vi "User mangement.vi"() -> ()   [LabVIEW 2017]
uses:
  <vilib>/Utility/error.llb/DialogType.ctl
  <vilib>/addons/database/Connection.llb/DB Tools Open Connec (Path).vi
  <vilib>/addons/database/NI_Database_API.lvlib
panel:
  in  "NEW":bool
  in  "DELETE":bool
  out "error out":errorcluster
  in  "error in (no error)":errorcluster
  in  "EXIT":bool
  in  "SAVE":bool
  in  "Authority":string(combo)
  in  "re_enter password":string
  in  "Password":string
  in  "NAME":string(combo)
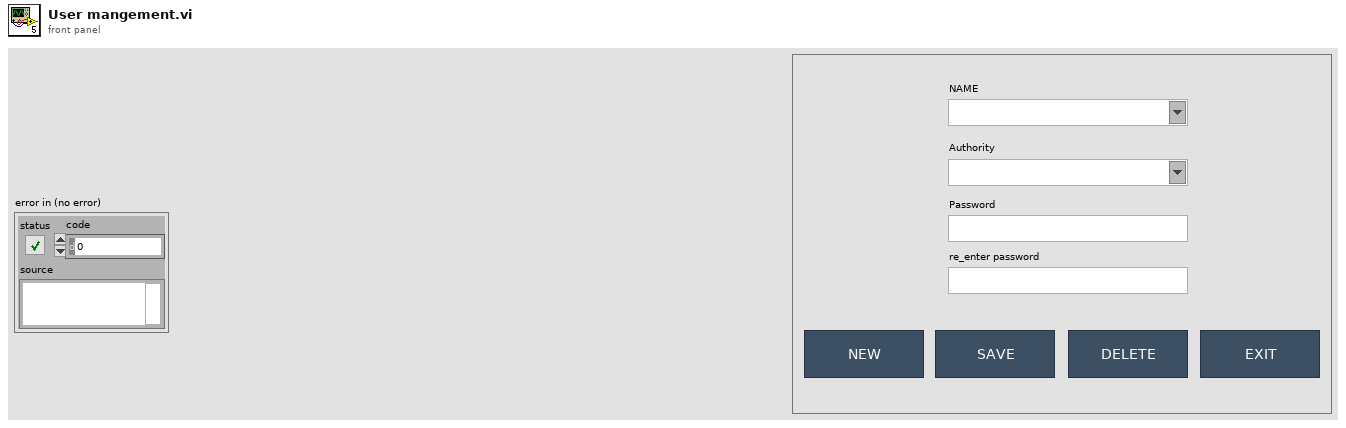
[diagram p1: front panel]
types:
  T1 = typedef "DialogType.ctl" = u16
  T2 = typedef "NI_Database_API.lvlib/Conn ObjectReference.ctl" = refnum<k1>
  T3 = cluster{"NAME":string, "Authority":string, "Password":string, "re_enter password":string}
  T4 = enum32{"invalid app kind", "Development System", "Run Time System", "Student Edition", "Embedded LabVIEW", "Evaluation", "Custom"}
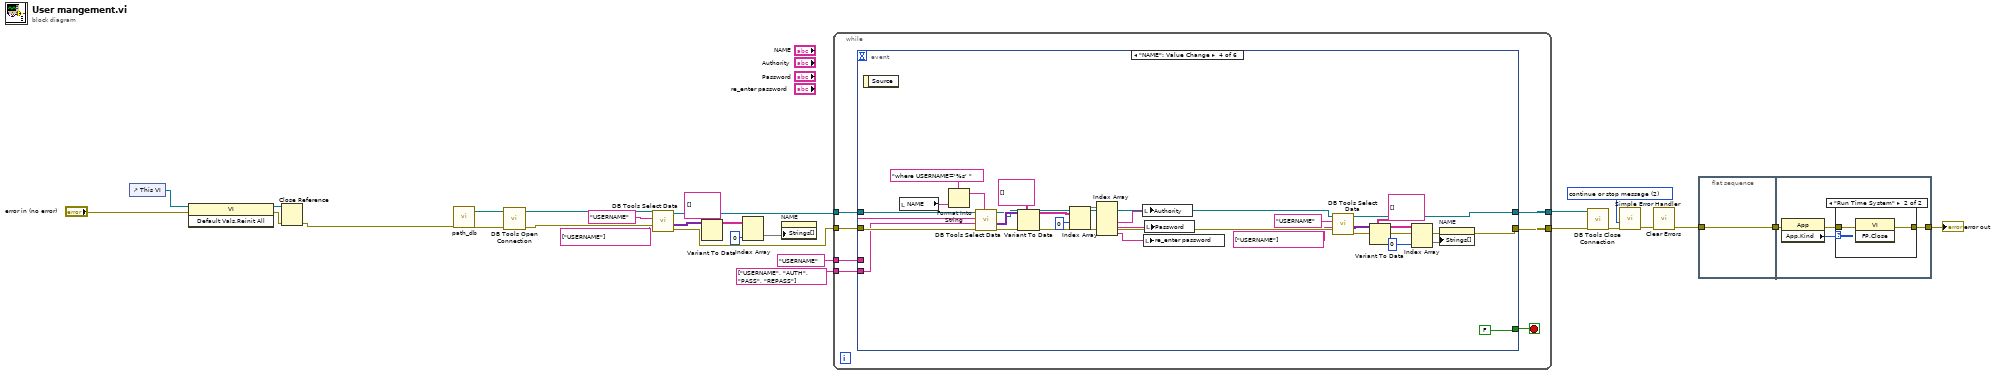
[diagram p0: block diagram]
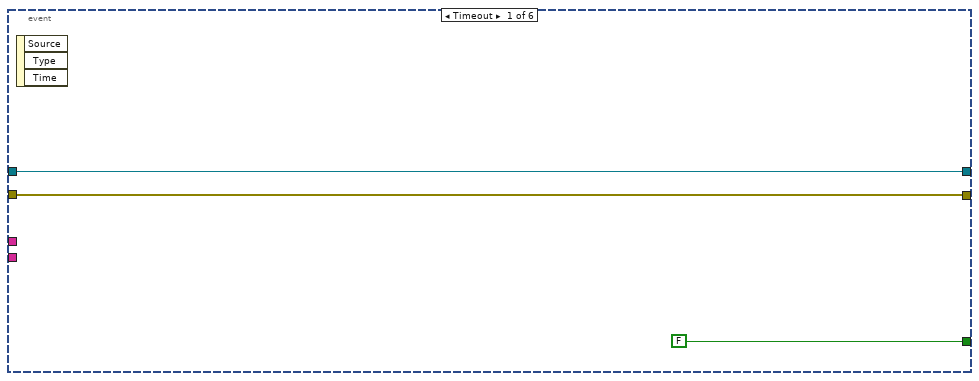
[diagram p3: hidden frame]
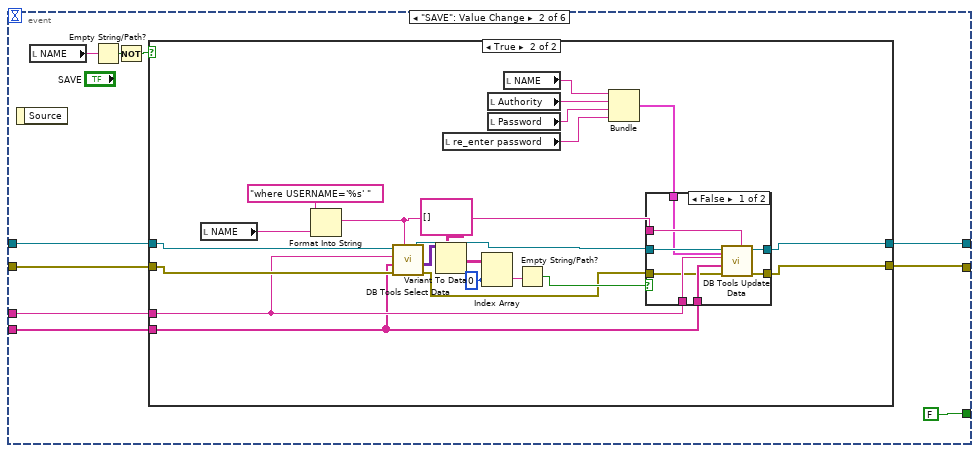
[diagram p4: hidden frame]
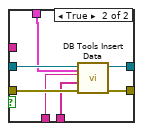
[diagram p6: hidden frame]
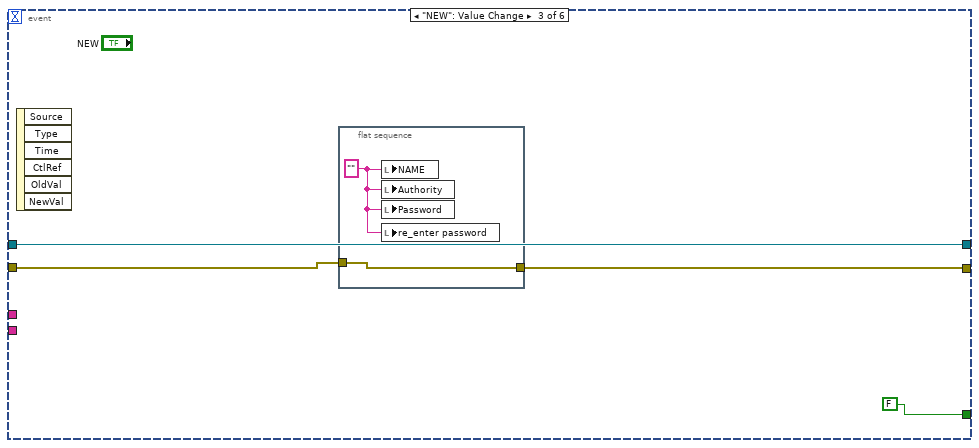
[diagram p7: hidden frame]
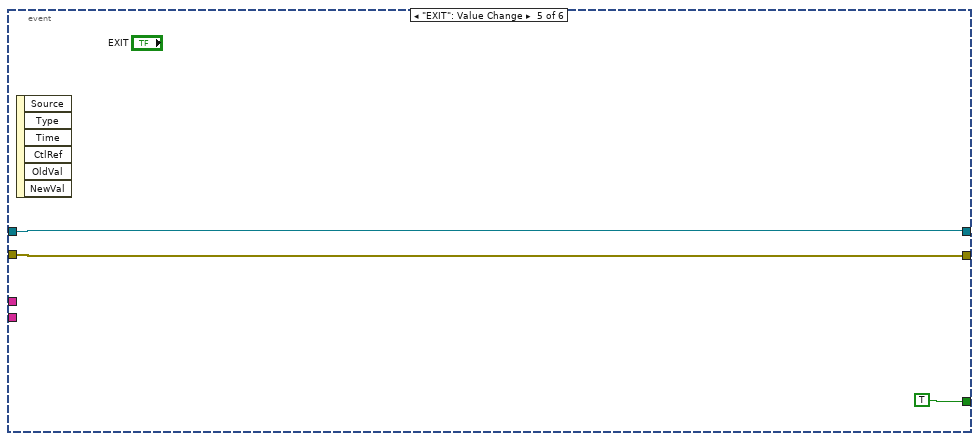
[diagram p8: hidden frame]
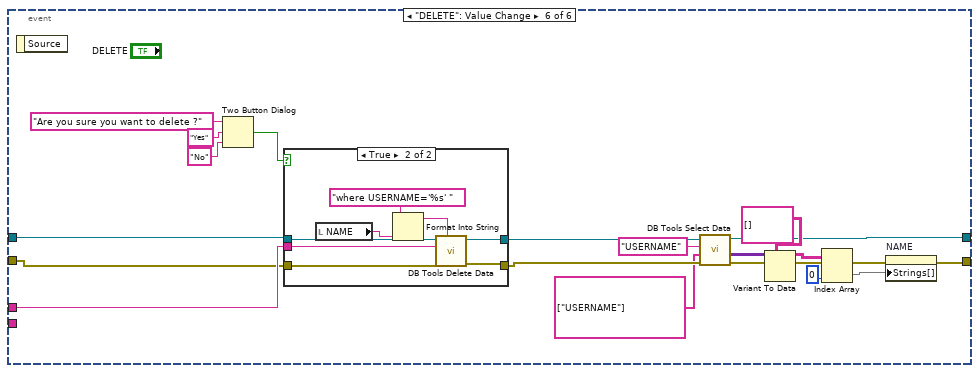
[diagram p9: hidden frame]
diagram:
  w10 = T1 2 items=["no dialog", "OK message", "continue or stop message", "OK message + warnings", "continue/stop + warnings"] ("type of dialog (OK msg:1)")
  n1 = control-ref of="This VI"() -> (w28:refnum<vi>)
  n2 = invoke class="VI" method="Default Vals.Reinit All"(reference=w28, error in="error in (no error)") -> (reference out=w26:refnum<vi>, error out=w27:errorcluster)  [unwired: 1 in, 1 out]
  n3 = Close Reference(reference=w26, error in (no error)=w27) -> (error out=w1:errorcluster)
  n4 = call "path_db.vi"("error in"=w1) -> ("error out"=w3:errorcluster, "resulting string"=w2:path)  [unwired: 9 in]
  n5 = call-poly <vilib>:"DB Tools Open Connection.vi"("error in (no error)"=w3, "connection information"=w2) -> ("error out"=w17:errorcluster, "connection reference"=w19:T2)  [unwired: 6 in]
  n6 = call <vilib>:"DB Tools Select Data.vi"("error in (no error)"=w17, "columns"=string[] ["USERNAME"], "table"="USERNAME", "connection reference"=w19) -> ("error out"=w16:errorcluster, "data"=w23:variant[][], "connection reference out"=w18:T2)  [unwired: 2 in]
  n7 = Variant To Data(type=string[][] [], Variant=w23) -> (data=w20:string[][])  [unwired: 1 in, 1 out]
  n8 = Index Array(array=w20, index (col)=0 ("disabled index (col)")) -> (element=w15:string[])  [unwired: 1 in]
  n9 = property on="NAME" class="CmbBox"("Strings[]"=w15) -> ()  [unwired: 2 in, 2 out]
  n10 = while {
    tunnel: w16 -> [w34]
    tunnel: [w33] -> w8
    tunnel: w18 -> [w32]
    tunnel: [w31] -> w7
    tunnel: "USERNAME" ("table") -> [w30]
    tunnel: string[] ["USERNAME", "AUTH", "PASS", "REPASS"] -> [w29]
    stop <- w35 stop-if-true
    n11 = event shown="[3] \"NAME\": Value Change" {
      selector: _ -> [_ _ _ _ _ _]
      dyn-events: _ -> [_ _ _ _ _ _]
      timeout: _ -> [_ _ _ _ _ _]
      tunnel: [FALSE FALSE FALSE FALSE TRUE _] -> w35
      tunnel: w34 -> [w36 w44 w89 w113 w122 w127]
      tunnel: [w36 w43 w88 w97 w122 w126] -> w33
      tunnel: w32 -> [w37 w42 w91 w114 w123 w129]
      tunnel: [w37 w41 w91 w95 w123 w128] -> w31
      tunnel: w30 -> [_ w39 _ w112 _ w130]
      tunnel: w29 -> [_ w40 _ w111 _ _]
      event Timeout {
        n12 = event-data() -> ()  [unwired: 1 in, 3 out]
      }
      event "SAVE": Value Change {
        n13 = event-data() -> ()  [unwired: 1 in, 1 out]
        n14 = local read "NAME"() -> (w46:string)
        n15 = Empty String/Path?(string/path=w46) -> (empty?=w47:bool)
        n16 = Not(x=w47) -> (.not. x?=w45:bool)
        n17 = case shown="True" w45 {
          tunnel: w44 -> [w49 w61]
          tunnel: [w49 w62] -> w43
          tunnel: w42 -> [w50 w59]
          tunnel: [w50 w60] -> w41
          tunnel: w40 -> [_ w57]
          tunnel: w39 -> [_ w58]
          frame False {
          }
          frame True {
            w65 = 0 ("disabled index (col)")
            n18 = local read "NAME"() -> (w51:string)
            n19 = Format Into String(format string="where USERNAME='%s' ", w51) -> (resulting string=w71:string)  [unwired: 2 in, 1 out]
            n20 = call <vilib>:"DB Tools Select Data.vi"("condition"=w71, "error in (no error)"=w61, "columns"=w57, "table"=w58, "connection reference"=w59) -> ("error out"=w69:errorcluster, "data"=w67:variant[][], "connection reference out"=w70:T2)  [unwired: 1 in]
            n21 = Variant To Data(type=string[][] [], Variant=w67) -> (data=w66:string[][])  [unwired: 1 in, 1 out]
            n22 = local read "re_enter password"() -> (w52:string)
            n23 = Index Array(array=w66, index (row)=w65, index (col)=w65) -> (element=w68:string)
            n24 = local read "Authority"() -> (w54:string)
            n25 = local read "Password"() -> (w53:string)
            n26 = local read "NAME"() -> (w55:string)
            n27 = Empty String/Path?(string/path=w68) -> (empty?=w72:bool)
            n28 = Bundle("NAME"=w55, "Authority"=w54, "Password"=w53, "re_enter password"=w52) -> (w56:T3)  [unwired: 1 in]
            n29 = case shown="False" w72 {
              tunnel: [w73 w87] -> w62
              tunnel: [w79 w86] -> w60
              tunnel: w69 -> [w74 w85]
              tunnel: w70 -> [w80 w84]
              tunnel: w56 -> [w77 w83]
              tunnel: w58 -> [w76 w82]
              tunnel: w57 -> [w75 w81]
              tunnel: w71 -> [w78 _]
              frame False {
                n30 = call <vilib>:"DB Tools Update Data.vi"("condition"=w78, "data"=w77, "error in (no error)"=w74, "columns"=w75, "table"=w76, "connection reference"=w80) -> ("error out"=w73:errorcluster, "connection reference out"=w79:T2)  [unwired: 4 in]
              }
              frame True {
                n31 = call <vilib>:"DB Tools Insert Data.vi"("data"=w83, "error in (no error)"=w85, "columns"=w81, "table"=w82, "connection reference"=w84) -> ("error out"=w87:errorcluster, "connection reference out"=w86:T2)  [unwired: 5 in]
              }
            }
          }
        }
      }
      event "NEW": Value Change {
        n32 = event-data() -> ()  [unwired: 1 in, 6 out]
        n33 = flat-sequence {
          tunnel: w89 -> [w92]
          tunnel: [w92] -> _
          tunnel: [w92] -> w88
          frame #0 {
            w93 = ""
            n34 = local write "NAME"(w93) -> ()
            n35 = local write "Authority"(w93) -> ()
            n36 = local write "Password"(w93) -> ()
            n37 = local write "re_enter password"(w93) -> ()
          }
        }
      }
      event "NAME": Value Change {
        n38 = event-data() -> ()  [unwired: 1 in, 1 out]
        n39 = local read "NAME"() -> (w117:string)
        n40 = Format Into String(format string="where USERNAME='%s' ", w117) -> (resulting string=w120:string)  [unwired: 2 in, 1 out]
        n41 = call <vilib>:"DB Tools Select Data.vi"("condition"=w120, "error in (no error)"=w113, "columns"=w111, "table"=w112, "connection reference"=w114) -> ("error out"=w118:errorcluster, "data"=w119:variant[][], "connection reference out"=w96:T2)  [unwired: 1 in]
        n42 = Variant To Data(error in=w118, type=string[][] [], Variant=w119) -> (data=w108:string[][], error out=w98:errorcluster)
        n43 = Index Array(array=w108, index (row)=0) -> (element=w110:string[])  [unwired: 1 in]
        n44 = Index Array(array=w110) -> (element #2=w105:string, element #3=w107:string, element #4=w106:string)  [unwired: 4 in, 1 out]
        n45 = local write "Authority"(w105) -> ()
        n46 = local write "re_enter password"(w106) -> ()
        n47 = local write "Password"(w107) -> ()
        n48 = call <vilib>:"DB Tools Select Data.vi"("error in (no error)"=w98, "columns"=string[] ["USERNAME"], "table"="USERNAME", "connection reference"=w96) -> ("error out"=w97:errorcluster, "data"=w104:variant[][], "connection reference out"=w95:T2)  [unwired: 2 in]
        n49 = Variant To Data(type=string[][] [], Variant=w104) -> (data=w103:string[][])  [unwired: 1 in, 1 out]
        n50 = Index Array(array=w103, index (col)=0 ("disabled index (col)")) -> (element=w102:string[])  [unwired: 1 in]
        n51 = property on="NAME" class="CmbBox"("Strings[]"=w102) -> ()  [unwired: 2 in, 2 out]
      }
      event "EXIT": Value Change {
        n52 = event-data() -> ()  [unwired: 1 in, 6 out]
      }
      event "DELETE": Value Change {
        n53 = event-data() -> ()  [unwired: 1 in, 1 out]
        n54 = Two Button Dialog(message="Are you sure you want to delete ?", 1:"No" ("F button name (\"Cancel\")"), 2:"Yes" ("T button name (\"OK\")")) -> (T button?=w138:bool)
        n55 = case shown="True" w138 {
          tunnel: w127 -> [w144 w148]
          tunnel: [w144 w147] -> w142
          tunnel: w129 -> [w143 w150]
          tunnel: [w143 w149] -> w141
          tunnel: w130 -> [_ w146]
          frame False {
          }
          frame True {
            n56 = local read "NAME"() -> (w145:string)
            n57 = Format Into String(format string="where USERNAME='%s' ", w145) -> (resulting string=w152:string)  [unwired: 2 in, 1 out]
            n58 = call <vilib>:"DB Tools Delete Data.vi"("condition"=w152, "error in (no error)"=w148, "table"=w146, "connection reference"=w150) -> ("error out"=w147:errorcluster, "connection reference out"=w149:T2)  [unwired: 6 in]
          }
        }
        n59 = call <vilib>:"DB Tools Select Data.vi"("error in (no error)"=w142, "columns"=string[] ["USERNAME"], "table"="USERNAME", "connection reference"=w141) -> ("error out"=w126:errorcluster, "data"=w139:variant[][], "connection reference out"=w128:T2)  [unwired: 2 in]
        n60 = Variant To Data(type=string[][] [], Variant=w139) -> (data=w140:string[][])  [unwired: 1 in, 1 out]
        n61 = Index Array(array=w140, index (col)=0 ("disabled index (col)")) -> (element=w125:string[])  [unwired: 1 in]
        n62 = property on="NAME" class="CmbBox"("Strings[]"=w125) -> ()  [unwired: 2 in, 2 out]
      }
    }
  }
  n63 = call <vilib>:"DB Tools Close Connection.vi"("error in (no error)"=w8, "connection reference"=w7) -> ("error out"=w9:errorcluster)  [unwired: 5 in]
  n64 = call <vilib>:"Simple Error Handler.vi"("type of dialog (OK msg:1)"=w10, "error in (no error)"=w9) -> ("error out"=w13:errorcluster)  [unwired: 3 in, 4 out]
  n65 = call <vilib>:"Clear Errors.vi"("error in (no error)"=w13) -> ("error out"=w12:errorcluster)  [unwired: 5 in, 1 out]
  n66 = flat-sequence {
    tunnel: w12 -> [w153]
    tunnel: [w153] -> w14
    tunnel: [w154] -> w11
    tunnel: w14 -> [w155]
    frame #0 {
    }
    frame #1 {
      n67 = property class="App"(error in=w155) -> (error out=w156:errorcluster, "App.Kind"=w157:T4)  [unwired: 1 in, 1 out]
      n68 = case shown="\"Run Time System\"" w157 {
        tunnel: w156 -> [w158 w160]
        tunnel: [w158 w159] -> w154
        frame Default {
        }
        frame "Run Time System" {
          n69 = invoke class="VI" method="FP.Close"(error in=w160) -> (error out=w159:errorcluster)  [unwired: 2 in, 2 out]
        }
      }
    }
  }
  "error out" <- w11
